vi "Start.vi"(8 "error in (no error)":errorcluster, 10 "Target Time (seconds)":dbl, 11 "Timer in":refnum<class "Timer.lvclass">) -> (0 "error out":errorcluster, 3 "Timer DVR":refnum<data-value>)   [LabVIEW 2018, in "Timer.lvclass"]
uses:
  Timer.lvclass
  Timer.lvclass/Timer.ctl
  Set Target Time Elapsed Event.vi
  GUI.vi
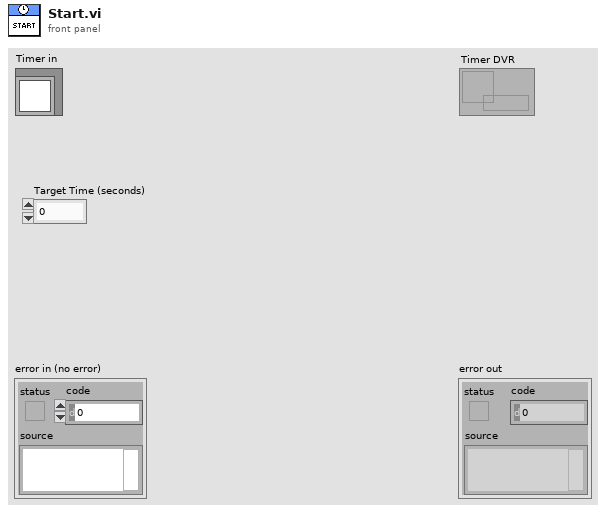
[diagram p1: front panel]
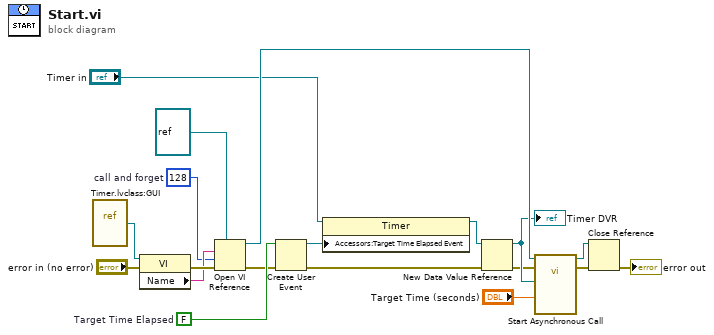
[diagram p0: block diagram]
diagram:
  w5 = FALSE  # Target Time Elapsed
  w12 = 128  # call and forget
  n1 = vi-ref "Timer.lvclass:GUI.vi"() -> (w17:refnum<vi>)
  n2 = property class="VI"(reference=w17, error in="error in (no error)") -> (error out=w19:errorcluster, "Name"=w18:string)  [unwired: 1 out]
  n3 = Open VI Reference(type specifier VI Refnum (for type only)=refnum<vi> refnum, vi path=w18, options=w12, error in (no error)=w19) -> (vi reference=w14:refnum<vi>, error out=w2:errorcluster)  [unwired: 2 in]
  n4 = Create User Event(user event datatype=w5, error in=w2) -> (user event=w3:refnum<user-event>, error out=w1:errorcluster)
  n5 = property class="Timer"(reference="Timer in", "Accessors:Target Time Elapsed Event"=w3) -> (reference out=w4:refnum<class "Timer.lvclass">)  [unwired: 1 in, 1 out]
  n6 = New Data Value Reference(data value=w4, error in=w1) -> (data value reference=w9:refnum<data-value>, error out=w6:errorcluster)
  "Timer DVR" <- w9
  n7 = call-by-ref "Start Asynchronous Call"(reference=w14, error in=w6, "Target Time (seconds)"="Target Time (seconds)", "Timer DVR"=w9) -> (reference out=w16:refnum<vi>, error out=w15:errorcluster)  [unwired: 10 in]
  n8 = Close Reference(reference=w16, error in (no error)=w15) -> (error out=→"error out":errorcluster)
